vi "Filter new data.vi"(7 "Headers":string[](array[string]), 8 "error in":errorcluster, 10 "Data IN":string[][](array[string]), 11 "Filter":refnum<vi>) -> (0 "error out":errorcluster, 3 "Filtered Array":string[][](array[string]))   [LabVIEW 2025, in "CAN-LIN Raw Bus Capture UI.lvlib"]
uses:
  CAN-LIN Raw Bus Capture UI.lvlib
  <vilib>/Utility/error.llb/whitespace.ctl
  <vilib>/Utility/error.llb/Trim Whitespace One-Sided.vi
  Table_Filtering/Table_Filtering.lvlib
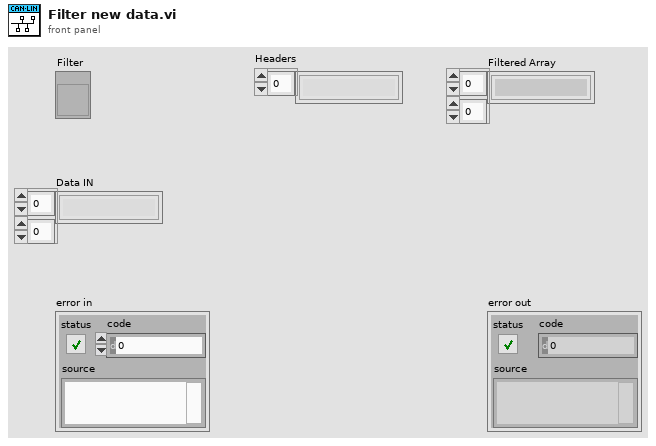
[diagram p1: front panel]
types:
  T1 = typedef "whitespace.ctl" = u16
  T2 = cluster{"FIELD":string, "OPERATOR":string, "VALUE":string}[]
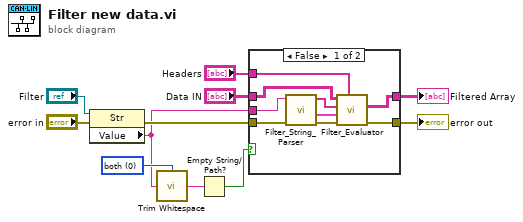
[diagram p0: block diagram]
diagram:
  w5 = T1 0 items=["both", "start of string", "end of string"] ("location (both)")
  n1 = property class="Str"(reference="Filter", error in="error in") -> (error out=w11:errorcluster, "Value"=w2:string)  [unwired: 1 out]
  n2 = call <vilib>:"Trim Whitespace.vi"("string"=w2, "location (both)"=w5) -> ("trimmed string"=w6:string)
  n3 = Empty String/Path?(string/path=w6) -> (empty?=w3:bool)
  n4 = case shown="False" w3 {
    tunnel: w11 -> [w20 w21]
    tunnel: [w19 w21] -> w8
    tunnel: "Data IN" -> [w17 w22]
    tunnel: [w14 w22] -> w4
    tunnel: w2 -> [w13 _]
    tunnel: "Headers" -> [w12 _]
    frame False {
      n5 = call "Filter_String_Parser.vi"("error in"=w20, "Filter String"=w13) -> ("error constant"=w18:errorcluster, "Comparators"=w15:T2, "Boolean Connectors"=w16:string[])  [unwired: 7 in]
      n6 = call "Filter_Evaluator.vi"("Headers"=w12, "Error"=w18, "Comparators"=w15, "Boolean Connectors"=w16, "Prefiltered Data"=w17) -> ("Error Out"=w19:errorcluster, "Filtered Array"=w14:string[][])  [unwired: 4 in, 1 out]
    }
    frame True {
    }
  }
  "error out" <- w8
  "Filtered Array" <- w4
